vi "Check Color.vi"(1 "Color in":T1=4914962) -> (21 "Color out":T1=4914962)   [LabVIEW 2020, in "lv_icon.lvlib"]
doc: "Check whether or not the color is the magic transparency color constant. If so, return RGB (246, 246, 246)."
uses:
  <vilib>/LabVIEW Icon API/lv_icon/lv_icon.lvlib
  <vilib>/LabVIEW Icon API/lv_icon/Controls/IEColor.ctl
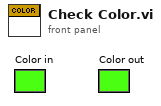
[diagram p1: front panel]
types:
  T1 = typedef "IEColor.ctl" = u32
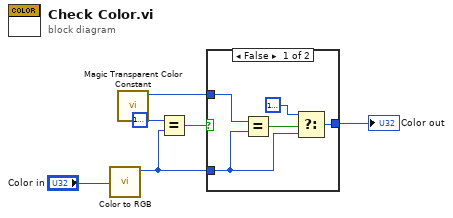
[diagram p0: block diagram]
diagram:
  n1 = call <vilib>:"Color to RGB.vi"("Color"="Color in") -> ("Resolved Color"=w1:u32)  [unwired: 3 out]
  n2 = call <vilib>:"Magic Transparent Color Constant.vi"() -> ("Magic transparent color constant"=w3:u32)  [unwired: 11 out]
  n3 = Equal?(x=T1 16777216, y=w1) -> (x = y?=w5:bool)
  n4 = case shown="False" w5 {
    tunnel: [w9 w12] -> w4
    tunnel: w3 -> [w11 w12]
    tunnel: w1 -> [w7 _]
    frame False {
      n5 = Equal?(x=w11, y=w7) -> (x = y?=w10:bool)
      n6 = Select(t=T1 16185078 ("x"), s=w10, f=w7) -> (s? t:f=w9:T1)
    }
    frame True {
    }
  }
  "Color out" <- w4
